vi "Operaciones Basicas.vi"() -> ()   [LabVIEW 2014]
panel:
  in  "stop":bool
  out "Division":dbl(slide) scale=0.0..10.0
  out "Multiplicacion":dbl(slide) scale=0.0..100.0
  out "Resta":dbl(slide) scale=-100.0..100.0
  out "Suma":dbl
  in  "Vertical Pointer Slide":dbl(slide) scale=0.0..100.0
  in  "Dial 2":dbl(knob) scale=0.0..10.0
  in  "Knob 2":dbl(knob) scale=0.0..10.0
  in  "Knob":dbl(knob) scale=0.0..10.0
  in  "Numeric":dbl
  in  "Dial":dbl(knob) scale=0.0..10.0
  in  "Slide":dbl(slide) scale=0.0..100.0
  in  "Numeric Control":dbl
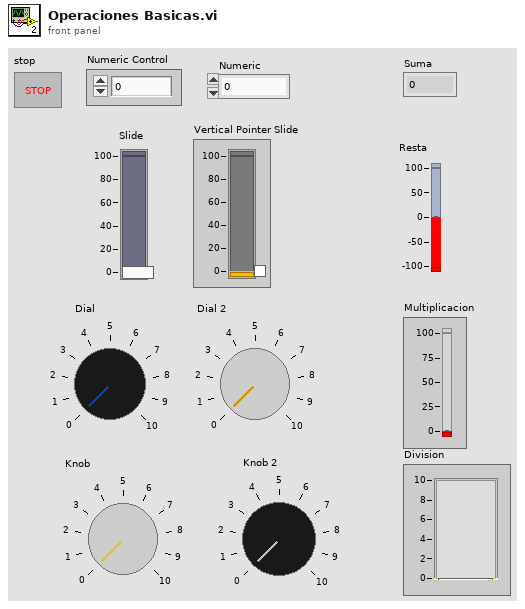
[diagram p1: front panel]
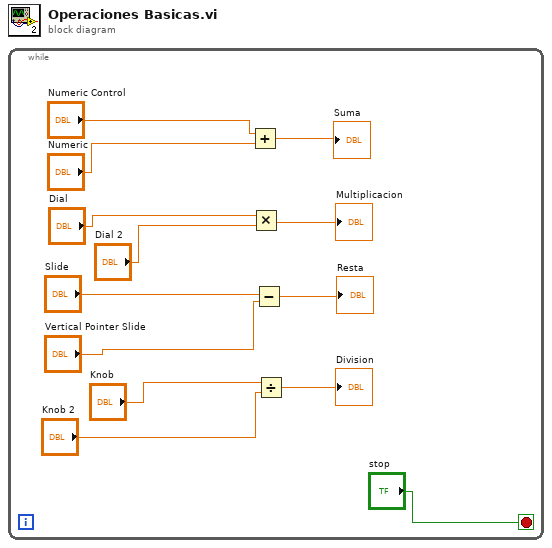
[diagram p0: block diagram]
diagram:
  n1 = while {
    stop <- "stop" stop-if-true
    n2 = Add(x="Numeric Control", y="Numeric") -> (x+y=→"Suma":dbl)
    n3 = Multiply(x="Dial", y="Dial 2") -> (x*y=→"Multiplicacion":dbl)
    n4 = Subtract(x="Slide", y="Vertical Pointer Slide") -> (x-y=→"Resta":dbl)
    n5 = Divide(x="Knob", y="Knob 2") -> (x/y=→"Division":dbl)
  }
